vi "Set-Frame-time.vi"(8 "error in (no error)":errorcluster, 9 "Frame rate":dbl caption="Frame rate [fps]", 10 "Frame time in":dbl caption="Frame time [s]", 11 "Camera in":refnum<class "Camera.lvclass">) -> (0 "error out":errorcluster, 2 "Frame time":dbl caption="Frame time [s]", 3 "Camera out":refnum<class "Camera.lvclass">)   [LabVIEW 2013, in "CameraVision.lvlib" / "Camera.lvclass"]
uses:
  Camera.lvclass
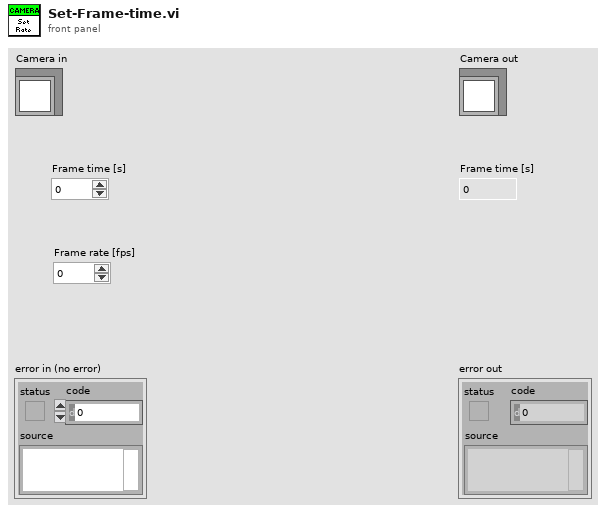
[diagram p1: front panel]
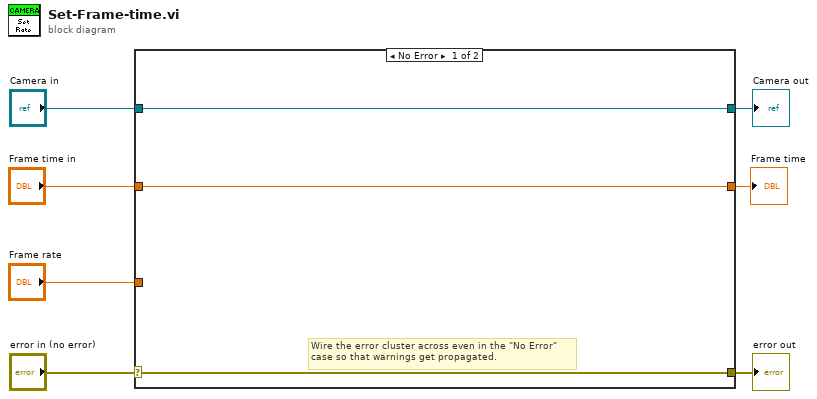
[diagram p0: block diagram]
diagram:
  n1 = case shown="No Error" "error in (no error)" {
    selector: "error in (no error)" -> [w9 w13]
    tunnel: [w9 w13] -> w6
    tunnel: [w10 w12] -> w4
    tunnel: "Camera in" -> [w10 w12]
    tunnel: "Frame rate" -> [_ _]
    tunnel: "Frame time in" -> [w8 w11]
    tunnel: [w8 w11] -> w1
    frame No Error {
      # "Wire the error cluster across even in the \"No Error\"\ncase so that warnings get propagated."
    }
    frame Error {
    }
  }
  "error out" <- w6
  "Camera out" <- w4
  "Frame time" <- w1
